vi "Create Data File.vi"(8 "error in (no error)":errorcluster caption="错误输入（无错误）", 10 "Acquisition and Logging Configuration":T1={"Data Rate (Hz)"=1.0, "Samples per Read"=0, "Number of Reads to Save"=0, "Data File Name"="", "TDMS Properties"=[], "Number of Channels"=4, "Channel Scale Array"=[0.0, 0.0, 0.0, 0.0], "Channel Names"=[], "Trigger - RMS Value"=0.0, "Trigger - Channel"=0, "Trigger - Time (Minute)"=0, "Enable RMS Trigger"=FALSE, "Enable Time Trigger"=FALSE, "Always Log"=FALSE} caption="采集与记录配置") -> (0 "error out":errorcluster caption="错误输出", 3 "TDMS File Reference":refnum<k34> caption="TDMS文件引用")   [LabVIEW 2013]
uses:
  controls/Acquisition and Logging Configuration.ctl
  controls/TDMS Properties.ctl
  Globals/Global - Configuration Options.vi
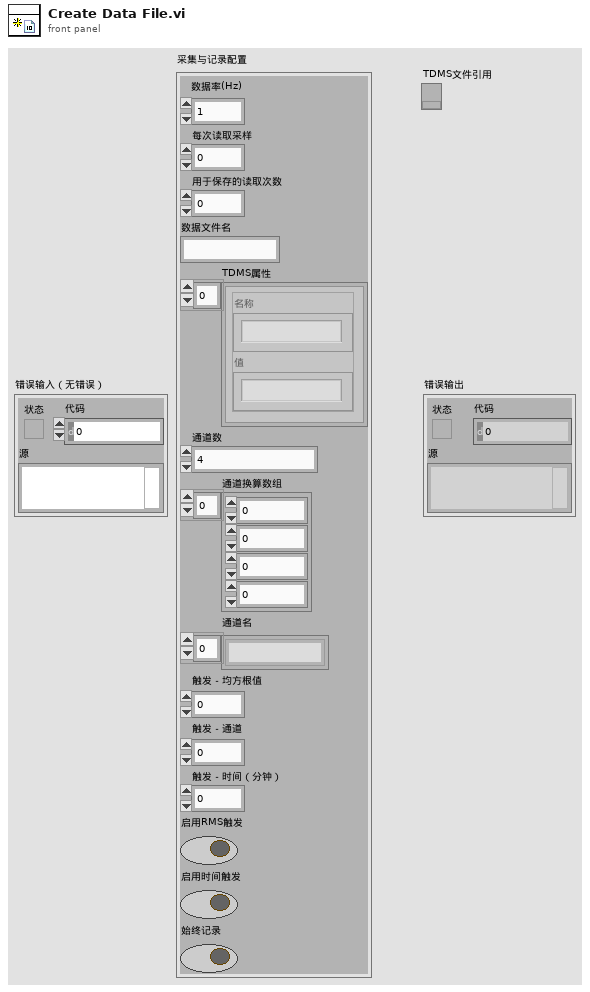
[diagram p1: front panel]
types:
  T1 = typedef "Acquisition and Logging Configuration.ctl" = cluster{"Data Rate (Hz)":dbl, "Samples per Read":i32, "Number of Reads to Save":i32, "Data File Name":string, "TDMS Properties":T2[], "Number of Channels":i32, "Channel Scale Array":dbl[], "Channel Names":string[], "Trigger - RMS Value":dbl, "Trigger - Channel":i32, "Trigger - Time (Minute)":i32, "Enable RMS Trigger":bool, "Enable Time Trigger":bool, "Always Log":bool}
  T2 = typedef "TDMS Properties.ctl" = cluster{"Name":string, "Value":string}
  T3 = enum16{"open", "open or create", "create or replace", "create", "open (read-only)"}
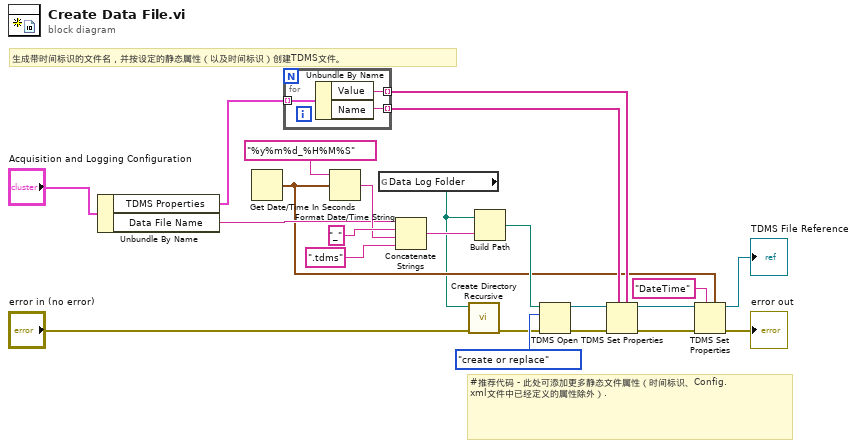
[diagram p0: block diagram]
diagram:
  # "生成带时间标识的文件名，并按设定的静态属性（以及时间标识）创建TDMS文件。"
  # "#推荐代码 - 此处可添加更多静态文件属性（时间标识、Config.xml文件中已经定义的属性除外）."
  n1 = Unbundle By Name("Acquisition and Logging Configuration") -> ("TDMS Properties"=w12:T2[], "Data File Name"=w18:string)
  n2 = Get Date/Time In Seconds() -> (seconds since 1Jan1904=w8:timestamp)
  n3 = for {
    tunnel: w12 -> [w26] mode=indexing
    tunnel: [w25] -> w11 mode=indexing
    tunnel: [w24] -> w10 mode=indexing
    n4 = Unbundle By Name(w26) -> ("Value"=w24:string, "Name"=w25:string)
  }
  n5 = Format Date/Time String(time format string (%c)="%y%m%d_%H%M%S", seconds (now)=w8) -> (date/time string=w22:string)  [unwired: 1 out]
  n6 = global read "Global - Configuration Options.vi" "Data Log Folder"() -> (w3:path)
  n7 = Concatenate Strings(w18, "_" ("string"), w22, ".tdms" ("string")) -> (w17:string)
  n8 = call <vilib>:"Create Directory Recursive.vi"("error in (no error)"="error in (no error)", "directory"=w3) -> ("error out"=w2:errorcluster)  [unwired: 3 in, 2 out]
  n9 = Build Path(base path=w3, name or relative path=w17) -> (appended path=w15:path)
  n10 = TDMS Open(8:w2, 10:T3."create or replace" ("operation (0:open)"), 11:w15) -> (0:w14:errorcluster, 3:w13:refnum<k34>)  [unwired: 4 in]
  n11 = TDMS Set Properties(5:w10, 7:w11, 8:w14, 11:w13) -> (0:w9:errorcluster, 3:w5:refnum<k34>)  [unwired: 2 in, 2 out]
  n12 = TDMS Set Properties(5:w8, 7:"DateTime" ("property names"), 8:w9, 11:w5) -> (0:→"error out":errorcluster, 3:→"TDMS File Reference":refnum<k34>)  [unwired: 2 in, 2 out]
